vi "Subvi hold HIGH.vi"(6 "Reset":bool, 9 "Input":bool) -> (1 "Output":bool)   [LabVIEW 2017]
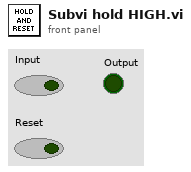
[diagram p1: front panel]
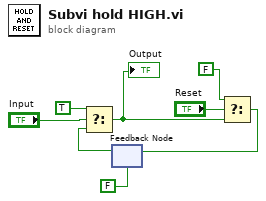
[diagram p0: block diagram]
diagram:
  n1 = feedback #1(FALSE) -> (w5:bool)
  n2 = Select(t=TRUE, s="Input", f=w5) -> (s? t:f=w1:bool)
  "Output" <- w1
  n3 = Select(t=FALSE, s="Reset", f=w1) -> (s? t:f=w4:bool)
  n4 = feedback-in #1(w4) -> ()
